vi "ascii to set of items.vi"(11 "ascii bytes":u8[](array[numeric])) -> (3 "set out":set{u8}(c389))   [LabVIEW 2019]
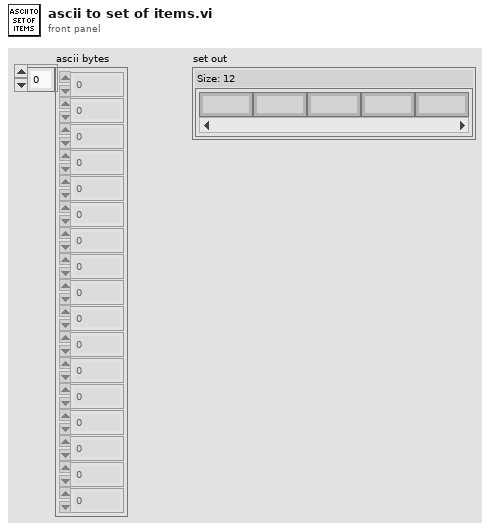
[diagram p1: front panel]
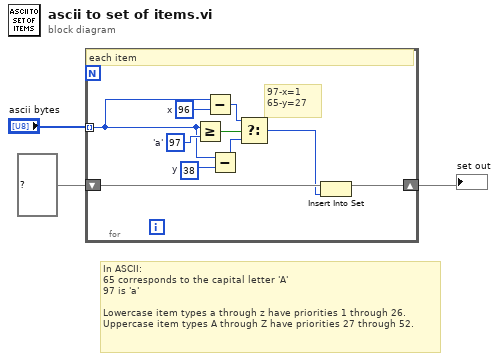
[diagram p0: block diagram]
diagram:
  # "In ASCII:\n65 corresponds to the capital letter 'A'\n97 is 'a'\n\nLowercase item types a through z have priorities 1 through 26.\nUppercase item types A through Z have priorities 27 through 52."
  n1 = for {
    tunnel: "ascii bytes" -> [w6] mode=indexing
    shift-right: [w8] -> w3
    shift-left: set{u8} {} ("set out") -> [w7]
    w5 = u8 96  # x
    w10 = u8 38  # y
    w11 = u8 97  # 'a'
    # "97-x=1\n65-y=27"
    # "each item"
    n2 = Greater Or Equal?(x=w6, y=w11) -> (x >= y?=w12:bool)
    n3 = Subtract(x=w6, y=w5) -> (x-y=w13:u8)
    n4 = Subtract(x=w6, y=w10) -> (x-y=w9:u8)
    n5 = Select(t=w13, s=w12, f=w9) -> (s? t:f=w4:u8)
    n6 = Insert Into Set(10:w4, 11:w7) -> (3:w8:set{u8})  [unwired: 1 out]
  }
  "set out" <- w3
